vi "Add Channel.vi"(4 "Property Values":variant[](array[variant]), 6 "Property names":string[](array[string]), 8 "error in (no error)":errorcluster, 9 "Channel Setting":T1={"IOType"=enum."Input", "DefaultValue"=[[0.0]], "Dimensions"={"Row"=1, "Column"=1}, "Units"="", "Description"="", "Faultable"=FALSE}, 10 "Channel Name":string, 11 "Section Reference in":u64 format="%.0x") -> (0 "error out":errorcluster, 1 "Newly Created?":bool, 2 "Channel Reference":u64 format="%.0x", 3 "Section Reference out":u64 format="%.0x")   [LabVIEW 2013, in "Hierarchy Framework.lvlib" / "Section.lvclass"]
doc: "Adds a channel to the device or device subsection specified by <B>Section Reference in</B>. If the <B>Channel Name</B> you specify already exists, this VI updates the <B>Channel</B> information (<B>IOType</B>, <B>Units</B>, etc.), properties."
uses:
  Section.lvclass
  Channel/Ctls/ChannelSetting.ctl
  Channel/Ctls/IOType.ctl
  Channel/Ctls/Dimensions.ctl
  Generic/Generic.lvclass
  Channel/Channel.lvclass
  Item/Item.lvclass
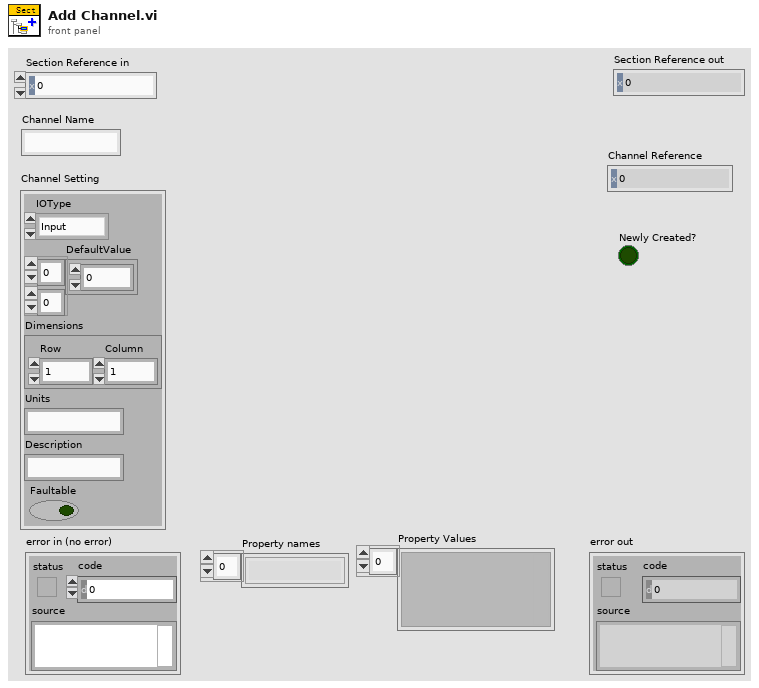
[diagram p1: front panel]
types:
  T1 = typedef "Hierarchy Framework.lvlib/Channel.lvclass/ChannelSetting.ctl" = cluster{"IOType":T2, "DefaultValue":dbl[][], "Dimensions":T3, "Units":string, "Description":string, "Faultable":bool}
  T2 = typedef "Hierarchy Framework.lvlib/Channel.lvclass/IOType.ctl" = enum16{"Input", "Output"}
  T3 = typedef "Hierarchy Framework.lvlib/Channel.lvclass/Dimensions.ctl" = cluster{"Row":i32, "Column":i32}
  T4 = typedef "Hierarchy Framework.lvlib/Item.lvclass/Item Reference.ctl" = u64
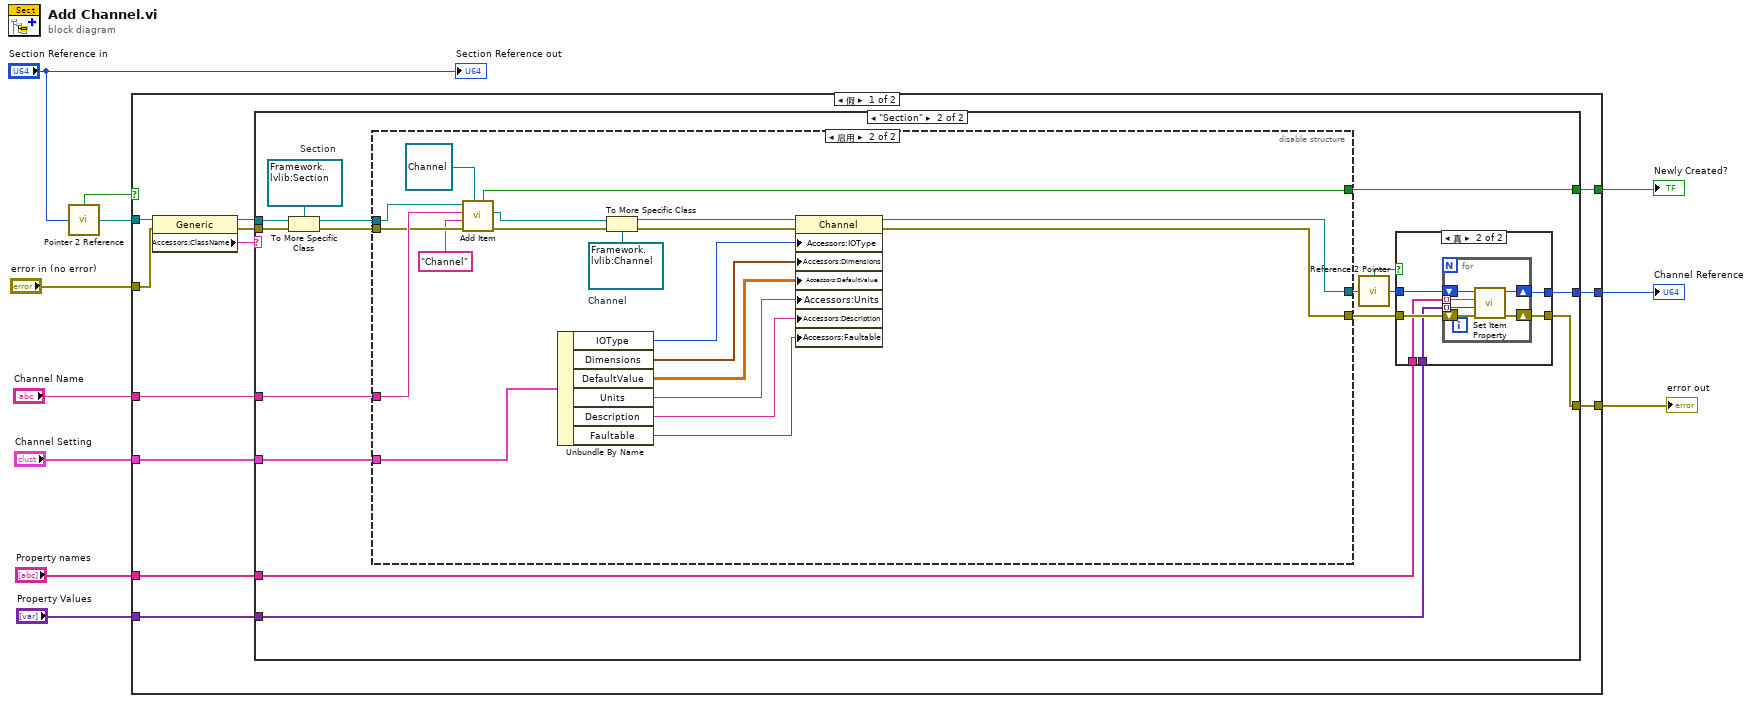
[diagram p0: block diagram]
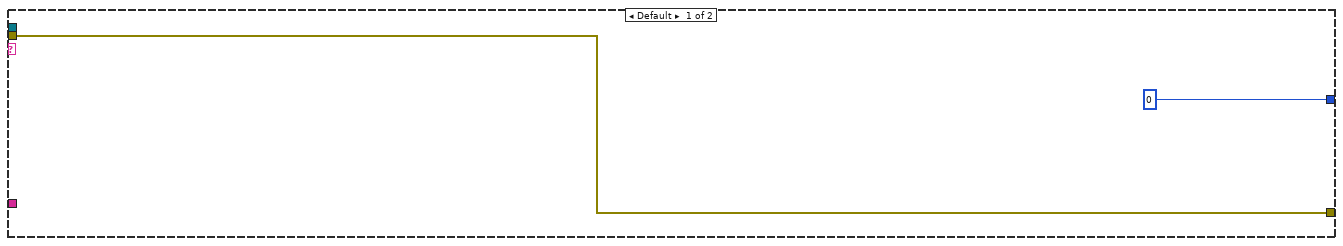
[diagram p2: hidden frame]
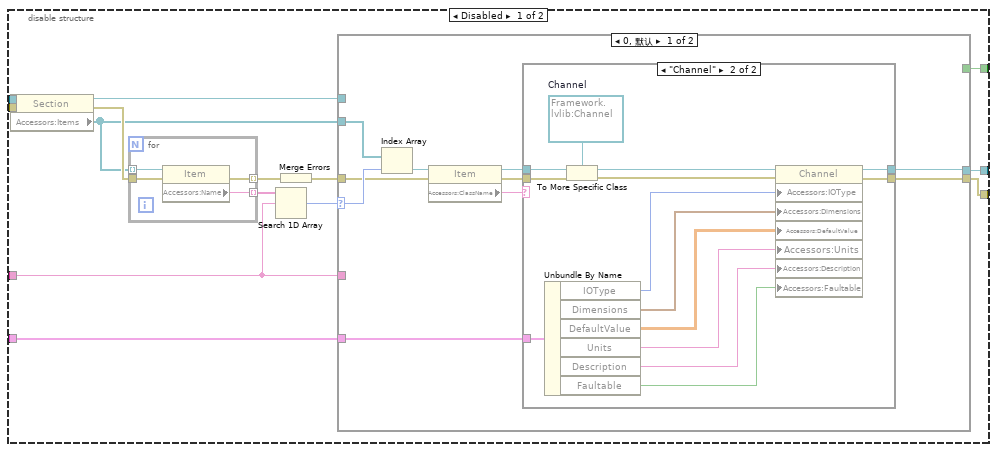
[diagram p3: hidden frame]
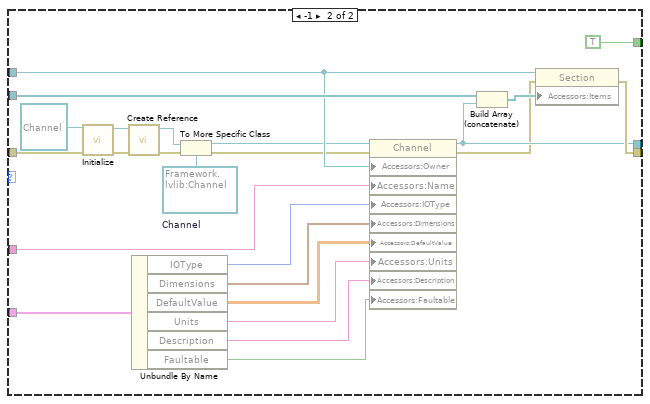
[diagram p5: hidden frame]
diagram:
  n1 = call "Pointer 2 Reference.vi"("Pointer"="Section Reference in") -> ("Not A Refnum?"=w5:bool, "Generic Reference"=w4:refnum<data-value>)
  n2 = case shown="假" w5 {
    tunnel: w4 -> [w19 _]
    tunnel: "Channel Name" -> [w23 _]
    tunnel: "error in (no error)" -> [w18 w144]
    tunnel: [w20 _] -> w9
    tunnel: [w22 _] -> w8
    tunnel: [w21 w144] -> w7
    tunnel: "Channel Setting" -> [w14 _]
    tunnel: "Property names" -> [w13 _]
    tunnel: "Property Values" -> [w12 _]
    frame False {
      n3 = property class="Generic"(reference=w19, error in=w18) -> (reference out=w16:refnum<data-value>, error out=w17:errorcluster, "Accessors:ClassName"=w15:string)
      n4 = case shown="\"Section\"" w15 {
        tunnel: w23 -> [_ w41]
        tunnel: [_ w40] -> w22
        tunnel: [w25 w29] -> w21
        tunnel: [u64 0 ("Pointer") w31] -> w20
        tunnel: w17 -> [w25 w35]
        tunnel: w16 -> [_ w34]
        tunnel: w14 -> [_ w33]
        tunnel: w13 -> [_ w28]
        tunnel: w12 -> [_ w27]
        frame Default {
        }
        frame "Section" {
          w39 = refnum<data-value> refnum  # Section
          n5 = To More Specific Class(target class=w39, reference=w34, error in=w35) -> (specific class reference=w38:refnum<data-value>, error out=w37:errorcluster)
          n6 = disable-structure shown="启用" {
            disable-tunnel: w41 -> [w48 w128]
            disable-tunnel: [w47 w112] -> w40
            disable-tunnel: w38 -> [w46 w129]
            disable-tunnel: w37 -> [w45 w127]
            disable-tunnel: [w44 w114] -> w36
            disable-tunnel: w33 -> [w43 w115]
            disable-tunnel: [w42 w113] -> w30
            frame Disabled {
              n7 = property class="Section"(reference=w46, error in=w45) -> (reference out=w50:refnum<data-value>, error out=w54:errorcluster, "Accessors:Items"=w49:refnum<data-value>[])
              n8 = for {
                tunnel: w49 -> [w109] mode=indexing
                tunnel: [w108] -> w55 mode=indexing
                tunnel: w54 -> [w107]
                tunnel: [w106] -> w53 mode=indexing
                n9 = property class="Item"(reference=w109, error in=w107) -> (error out=w106:errorcluster, "Accessors:Name"=w108:string)  [unwired: 1 out]
              }
              n10 = Search 1D Array(1D array=w55, element=w48) -> (index of element=w52:i32)  [unwired: 1 in]
              n11 = Merge Errors(w53) -> (w51:errorcluster)
              n12 = case shown="0, 默认" w52 {
                selector: w52 -> [w64 _]
                tunnel: w51 -> [w61 w100]
                tunnel: w50 -> [_ w96]
                tunnel: w49 -> [w65 w103]
                tunnel: w48 -> [_ w89]
                tunnel: [w63 w91] -> w44
                tunnel: [w56 w99] -> w42
                tunnel: [_ TRUE] -> w47
                tunnel: w43 -> [w57 w88]
                frame 0, Default {
                  n13 = Index Array(array=w65, index=w64) -> (element=w62:refnum<data-value>)
                  n14 = property class="Item"(reference=w62, error in=w61) -> (reference out=w59:refnum<data-value>, error out=w58:errorcluster, "Accessors:ClassName"=w60:string)
                  n15 = case shown="\"Channel\"" w60 {
                    tunnel: [w66 w69] -> w63
                    tunnel: w59 -> [w66 w80]
                    tunnel: w58 -> [w67 w79]
                    tunnel: w57 -> [_ w76]
                    tunnel: [w67 w68] -> w56
                    frame Default {
                    }
                    frame "Channel" {
                      w81 = refnum<data-value> refnum  # Channel
                      n16 = Unbundle By Name(w76) -> ("IOType"=w75:T2, "Dimensions"=w74:T3, "DefaultValue"=w73:dbl[][], "Units"=w72:string, "Description"=w71:string, "Faultable"=w70:bool)
                      n17 = To More Specific Class(target class=w81, reference=w80, error in=w79) -> (specific class reference=w78:refnum<data-value>, error out=w77:errorcluster)
                      n18 = property class="Channel"(reference=w78, error in=w77, "Accessors:IOType"=w75, "Accessors:Dimensions"=w74, "Accessors:DefaultValue"=w73, "Accessors:Units"=w72, "Accessors:Description"=w71, "Accessors:Faultable"=w70) -> (reference out=w69:refnum<data-value>, error out=w68:errorcluster)
                    }
                  }
                }
                frame -1 {
                  w102 = refnum<data-value> refnum  # Channel
                  n19 = call-dynamic "Initialize.vi"("error in (no error)"=w100, "Channel输入"=refnum<class "Channel.lvclass"> refnum ("Framework.lvlib:Channel")) -> ("error out"=w105:errorcluster, "Channel输出"=w104:refnum<class "Channel.lvclass">)  [unwired: 8 in]
                  n20 = call "Create Reference.vi"("error in (no error)"=w105, "Generic"=w104) -> ("error out"=w94:errorcluster, "Generic Reference"=w95:refnum<data-value>)  [unwired: 8 in]
                  n21 = Unbundle By Name(w88) -> ("IOType"=w87:T2, "Dimensions"=w86:T3, "DefaultValue"=w85:dbl[][], "Units"=w84:string, "Description"=w83:string, "Faultable"=w82:bool)
                  n22 = To More Specific Class(target class=w102, reference=w95, error in=w94) -> (specific class reference=w93:refnum<data-value>, error out=w92:errorcluster)
                  n23 = property class="Channel"(reference=w93, error in=w92, "Accessors:Owner"=w96, "Accessors:Name"=w89, "Accessors:IOType"=w87, "Accessors:Dimensions"=w86, "Accessors:DefaultValue"=w85, "Accessors:Units"=w84, "Accessors:Description"=w83, "Accessors:Faultable"=w82) -> (reference out=w91:refnum<data-value>, error out=w90:errorcluster)
                  n24 = Build Array (concatenate)(w103, w91) -> (w101:refnum<data-value>[])
                  n25 = property class="Section"(reference=w96, error in=w90, "Accessors:Items"=w101) -> (error out=w99:errorcluster)  [unwired: 1 out]
                }
              }
            }
            frame Enabled {
              w126 = refnum<data-value> refnum  # Channel
              n26 = call "Add Item.vi"("Type"=refnum<class "Channel.lvclass"> refnum ("Framework.lvlib:Channel"), "错误输入（无错误）"=w127, "TypeGUID"="Channel", "Name"=w128, "Section in"=w129) -> ("错误输出"=w116:errorcluster, "Item"=w117:refnum<data-value>, "Newly Created?"=w112:bool)  [unwired: 3 in, 1 out]
              n27 = Unbundle By Name(w115) -> ("IOType"=w123:T2, "Dimensions"=w122:T3, "DefaultValue"=w121:dbl[][], "Units"=w120:string, "Description"=w119:string, "Faultable"=w118:bool)
              n28 = To More Specific Class(target class=w126, reference=w117, error in=w116) -> (specific class reference=w125:refnum<data-value>, error out=w124:errorcluster)
              n29 = property class="Channel"(reference=w125, error in=w124, "Accessors:IOType"=w123, "Accessors:Dimensions"=w122, "Accessors:DefaultValue"=w121, "Accessors:Units"=w120, "Accessors:Description"=w119, "Accessors:Faultable"=w118) -> (reference out=w114:refnum<data-value>, error out=w113:errorcluster)
            }
          }
          n30 = call "Reference 2 Pointer.vi"("Generic Reference"=w36) -> ("Valid?"=w26:bool, "Pointer"=w32:u64)
          n31 = case shown="真" w26 {
            tunnel: w32 -> [w131 w137]
            tunnel: [w131 w136] -> w31
            tunnel: w30 -> [w130 w135]
            tunnel: [w130 w134] -> w29
            tunnel: w28 -> [_ w133]
            tunnel: w27 -> [_ w132]
            frame False {
            }
            frame True {
              n32 = for {
                shift-right: [w142] -> w136
                shift-left: w137 -> [w143]
                shift-right: [w140] -> w134
                shift-left: w135 -> [w141]
                tunnel: w133 -> [w139] mode=indexing
                tunnel: w132 -> [w138] mode=indexing
                n33 = call "Set Item Property.vi"("error in (no error)"=w141, "Value"=w138, "Property Name"=w139, "Item Reference in"=w143) -> ("error out"=w140:errorcluster, "Item Reference out"=w142:T4)  [unwired: 5 in, 1 out]
              }
            }
          }
        }
      }
    }
    frame True {
    }
  }
  "Channel Reference" <- w9
  "error out" <- w7
  "Newly Created?" <- w8
  "Section Reference out" <- "Section Reference in"
